vi "Camera.v10.vi"() -> ()   [LabVIEW 2015]
uses:
  Camera Properties.ctl
  Microscope Settings.ctl
  CameraState.ctl
  ModeEnum.ctl
  Stack_State.ctl
  Stack Track.ctl
  CameraControlTypeDef.ctl
  <vilib>/DAQmx/write.llb/DAQmx Write (Digital 1D Wfm NChan NSamp).vi
  <vilib>/DAQmx/write.llb/DAQmx Write (Analog 1D Wfm NChan NSamp).vi
  <vilib>/DAQmx/create/channels.llb/DAQmx Create Channel (DO-Digital Output).vi
  <vilib>/DAQmx/create/channels.llb/DAQmx Create Channel (AO-Voltage-Basic).vi
  <vilib>/Waveform/DWDTOps.llb/DWDT Append Digital Samples.vi
  <vilib>/Waveform/WDTOps.llb/WDT Append Waveforms DBL.vi
  <vilib>/Waveform/WDTOps.llb/WDT Number of Waveform Samples DBL.vi
  <vilib>/DAQmx/configure/timing.llb/DAQmx Timing (Sample Clock).vi
  <vilib>/Waveform/DWDTOps.llb/DWDT Uncompress Digital.vi
  <vilib>/DAQmx/miscellaneous.llb/DAQmx Fill In Error Info.vi
  <vilib>/vision/NI_Vision_Development_Module.lvlib
panel:
  in  "Tab Control":enum32{"Camera Settings", "Recording"}(tab)
  in  "Scans":dbl=1.0 min=0.0 max=10.0 step=0.05
  in  "?":bool
  in  "Microscope Settings":T1={"Mode"=enum."XY", "Slit"={"Scanning Mode"=12.0, "Slit Width /%"=5.0}, "Colour"=[{"Laser"=enum."561", "Filter"=4}], "Exposure/ms"=40.0, "Piezo Position /um"=0.0, "ROI"={"X"={"Start"=0.0, "Step"=1.0, "Range"=2048.0}, "Y"={"Start"=0.0, "Step"=1.0, "Range"=2048.0}, "Z "={"Start"=0.0, "Step"=1.0, "Range"=100.0}}, "Samples per millisecond"=100.0, "Relax/ms"=10.0, "Readout Direction"=2.0, "Trigger Source"=2.0, "Camera Delay /ms"=11.0, "Under Scan"=5.0} {"Under Scan" min=0.0 max=10.0 step=0.05; "ROI"."X"."Range" min=0.0 max=10.0 step=0.05; "ROI"."X"."Step" min=0.0 max=10.0 step=0.05; "ROI"."X"."Start" min=0.0 max=10.0 step=0.05; "ROI"."Y"."Range" min=0.0 max=10.0 step=0.05; "ROI"."Y"."Step" min=0.0 max=10.0 step=0.05; "ROI"."Y"."Start" min=0.0 max=10.0 step=0.05; "ROI"."Z"."Range" min=0.0 max=10.0 step=0.05; "ROI"."Z"."Step" min=0.0 max=10.0 step=0.05; "ROI"."Z"."Start" min=0.0 max=10.0 step=0.05; "Colour"."Filter" items=["Empty"=1, ""=2, ""=3, "561"=4, ""=5, "488"=6]; "Camera Delay /ms" min=0.0 max=10.0 step=0.05; "Trigger Source" items=["Internal"=1.0, "External"=2.0]; "Readout Direction" items=["Forward"=1.0, "Backward"=2.0]; "Slit"."Scanning Mode" items=["Full Frame"=1.0, "Slit Scanning"=12.0]; "Piezo Position /um" min=0.0 max=10.0 step=0.05}
  in  "Scan":bool
  in  "Scan Continuously":bool
  out "error IO":errorcluster
  in  "Advanced DCAM Controls":i32(listbox) caption="Multicolumn Listbox"
  in  "Properties":T2=4211904 items=["SENSOR MODE"=4212128, "CCD MODE"=4212384, "READOUT MODE"=4211872, "ACTIVE VIEW INDEX"=4343136, "BITS PER CHANNEL"=4342976, "IMAGE PIXEL TYPE"=4343296, "BINNING"=4215968, "EXPOSURE TIME"=2049184, "CONTRAST GAIN"=3163312, "CONTRAST OFFSET"=3163328, "LIGHT MODE"=2114720, "SENSITIVITY"=2114992, "PHOTON IMAGING MODE"=2115200, "HIGH DYNAMIC RANGE MODE"=3163360, "WHITE BALANCE"=3163568, "TEMPERATURE"=2115232, "TEMPERATURE TARGET"=2115264, "SENSOR COOLER FAN"=2115296, "LINEBUNDLE HEIGHT"=4212192, "MECHANICAL SHUTTER"=2115488, "BACK FOCUS POSITION"=8422304, "TRIGGER CONNECTOR"=1066432, "TRIGGER SOURCE"=1066144, "OUTPUT TRIGGER SOURCE"=1852576, "TRIGGER GLOBAL EXPOSURE"=2049680, "FIRST TRIGGER BEHAVIOR"=2049696, "CHANNEL SYNC"=1852352, "READOUT DIRECTION"=4211904, "PRE HSYNC COUNT"=1852704, "INTERNAL LINE SPEED"=4191408, "INTERNAL LINE INVERVAL"=4191424]
  in  "Multicolumn Listbox":i32(listbox)
  out "Image":T3(plugin-control)
  out "Histogram":T4(graph)
  in  "stop":bool
  in  "Signals Debugger":bool
  in  "Calibration":bool
  in  "MultiD Scan":bool
  in  "Stage Controller":bool
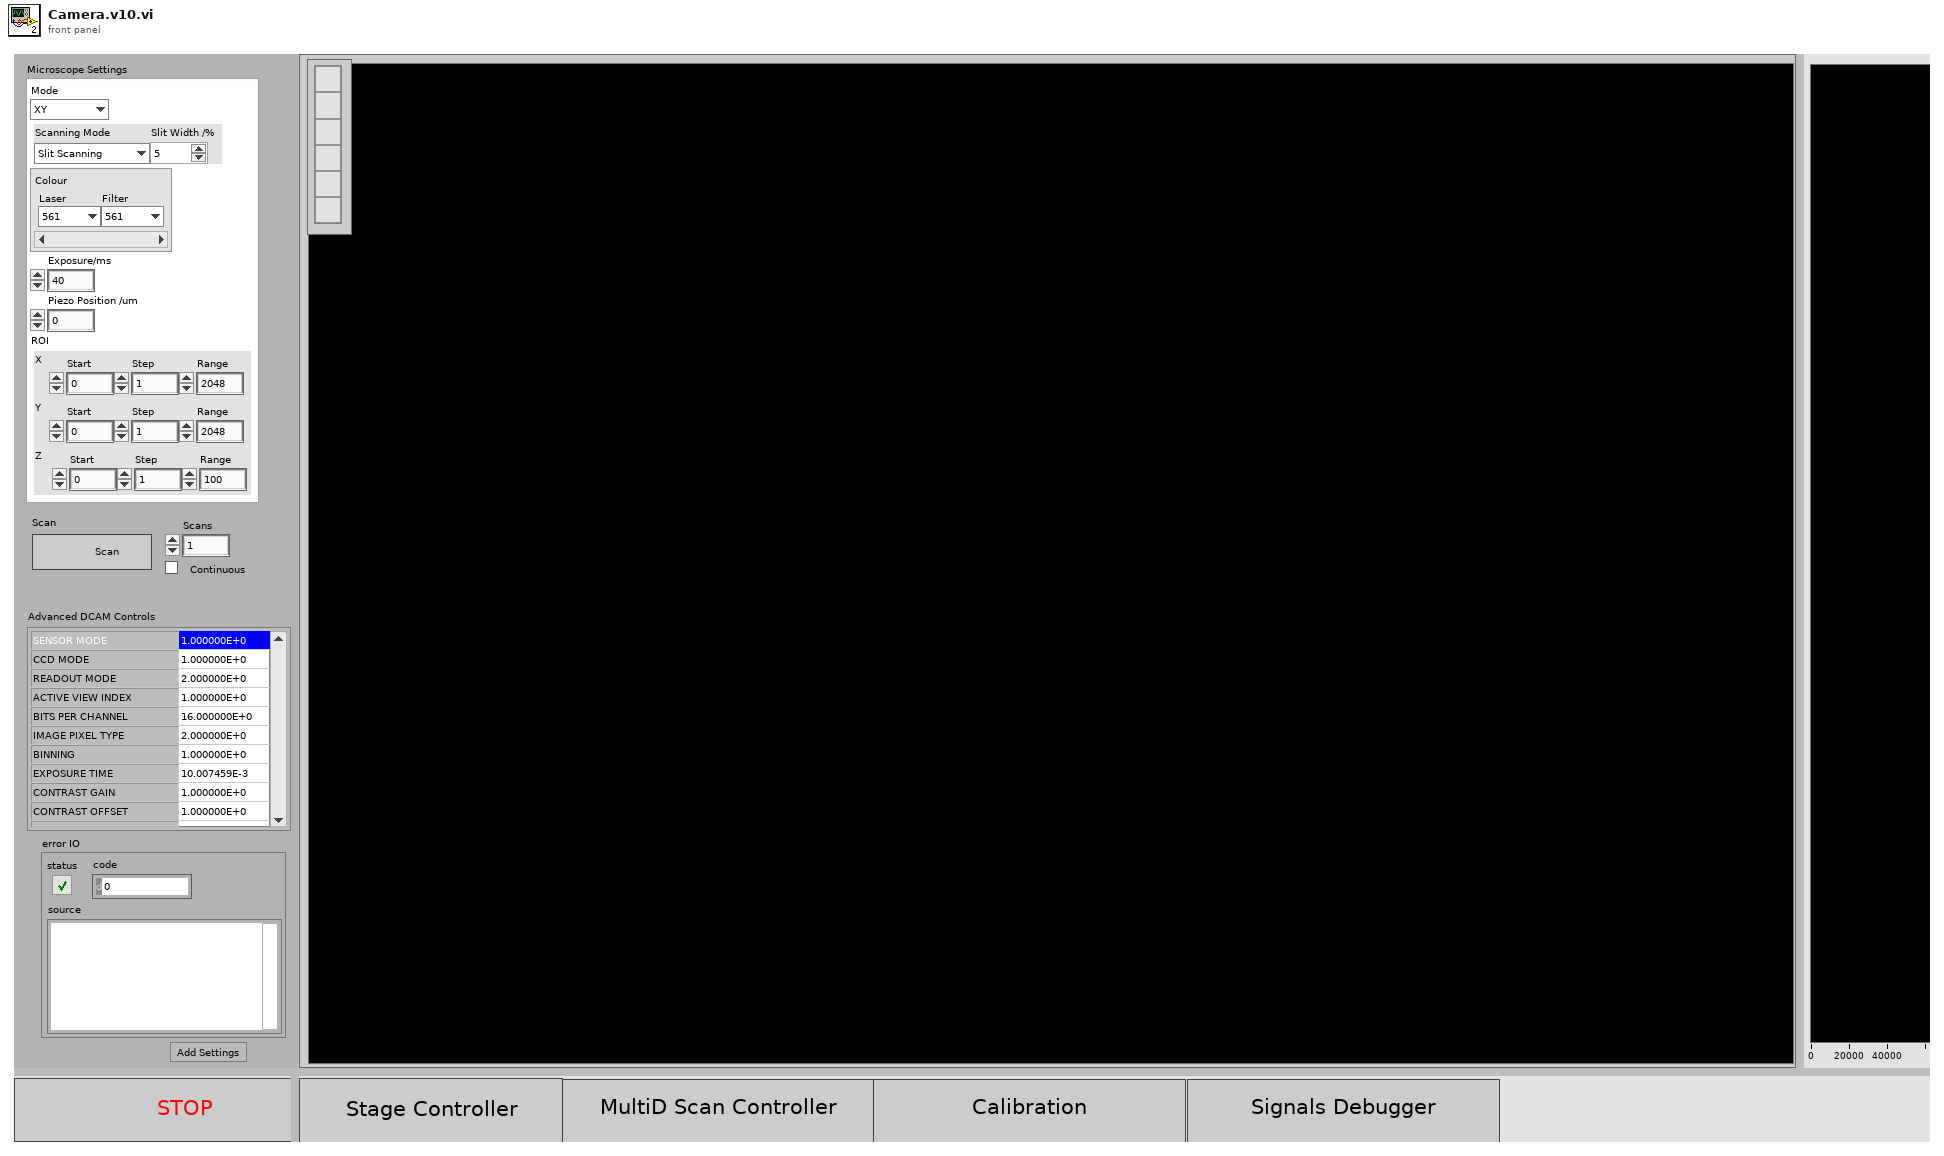
[diagram p1: front panel]
types:
  T1 = typedef "Microscope Settings.ctl" = cluster{"Mode":enum16{"X", "XY", "XYZ", "XYZT", "XYZC"}, "Slit":cluster{"Scanning Mode":dbl, "Slit Width /%":dbl}, "Colour":cluster{"Laser":enum16{"Brightfield", "445", "488", "561", "647"}, "Filter":u16}[], "Exposure/ms":dbl, "Piezo Position /um":dbl, "ROI":cluster{"X":cluster{"Start":dbl, "Step":dbl, "Range":dbl}, "Y":cluster{"Start":dbl, "Step":dbl, "Range":dbl}, "Z ":cluster{"Start":dbl, "Step":dbl, "Range":dbl}}, "Samples per millisecond":dbl, "Relax/ms":dbl, "Readout Direction":dbl, "Trigger Source":dbl, "Camera Delay /ms":dbl, "Under Scan":dbl}
  T2 = typedef "Camera Properties.ctl" = u32
  T3 = typedef "IMAQ Image.ctl" = refnum<image>
  T4 = cluster{"Starting Value":sgl, "Incremental Value":sgl, "Histogram":u32[]}
  T5 = cluster{"height":u32, "width":u32, "datatype":u32}
  T6 = typedef "CameraState.ctl" = enum16{"init", "active", "deinit"}
  T7 = typedef "ModeEnum.ctl" = enum16{"Idle", "generateWaves", "runWaves", "stop"}
  T8 = typedef "CameraControlTypeDef.ctl" = enum16{"Idle", "IntervalLineInt", "Ram Record", "HardDisk Record", "Disengage Update", "Update", "ROI", "Binning", "Scan Mode", "Trigger Mode", "Readout Mode", "Readout Direction", "Preview", "ROIWindow", "Trigger Source"}
  T9 = cluster{"Mode":u32, "Polarity":u32, "Times":u32, "Delay":dbl}
  T10 = typedef "Stack_State.ctl" = cluster{"State":T11, "Stack Number":i32, "Image":u16[][], "Stacks":i32}
  T11 = typedef "Stack Track.ctl" = enum16{"Idle", "Display", "Start Sequence", "Read Disk", "STOP", "Collecting", "End"}
  T12 = enum32{"Invalid", "Standard", "Closed", "Hidden", "Minimized", "Maximized"}
  T13 = typedef "Image Type" = u32
  T14 = cluster{"Analogue Out":waveform(dbl)[], "Digital Out":digitalwaveform[]}
  T15 = cluster{"State":T11, "Timeout":i32, "Data 16":u16[][], "Timeout":i32}
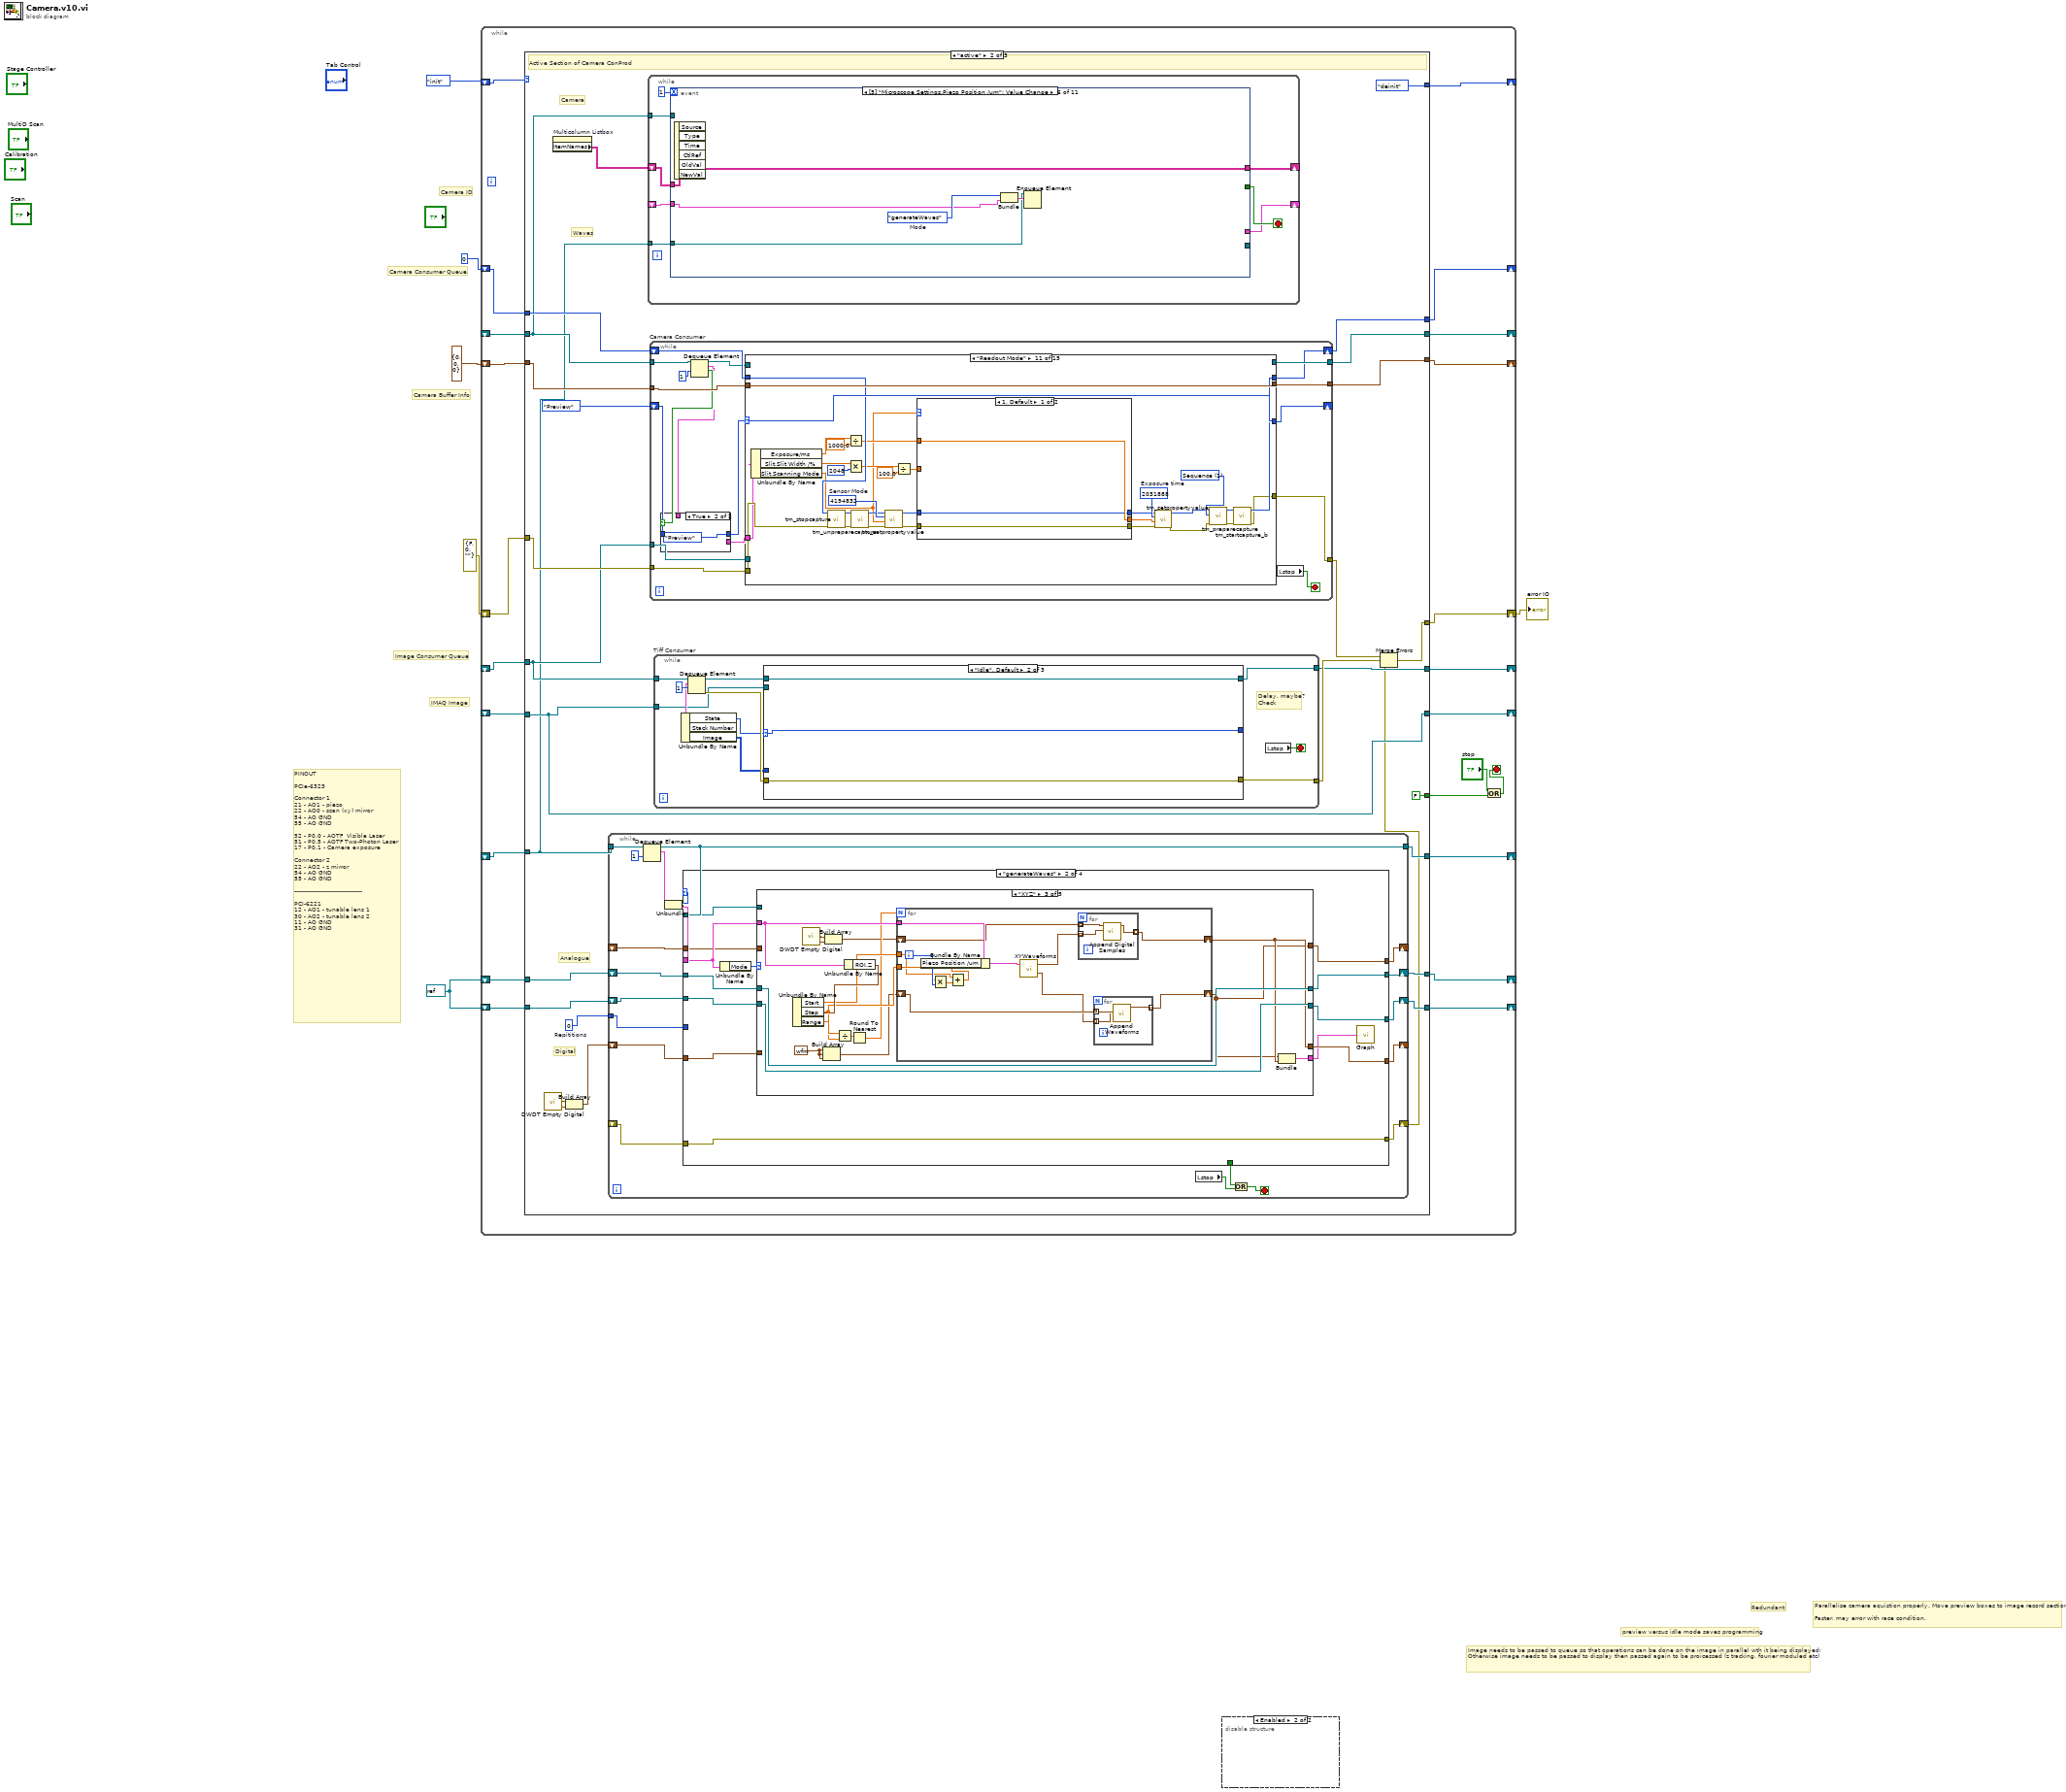
[diagram p0: block diagram]
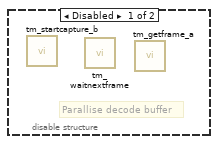
[diagram p2: hidden frame]
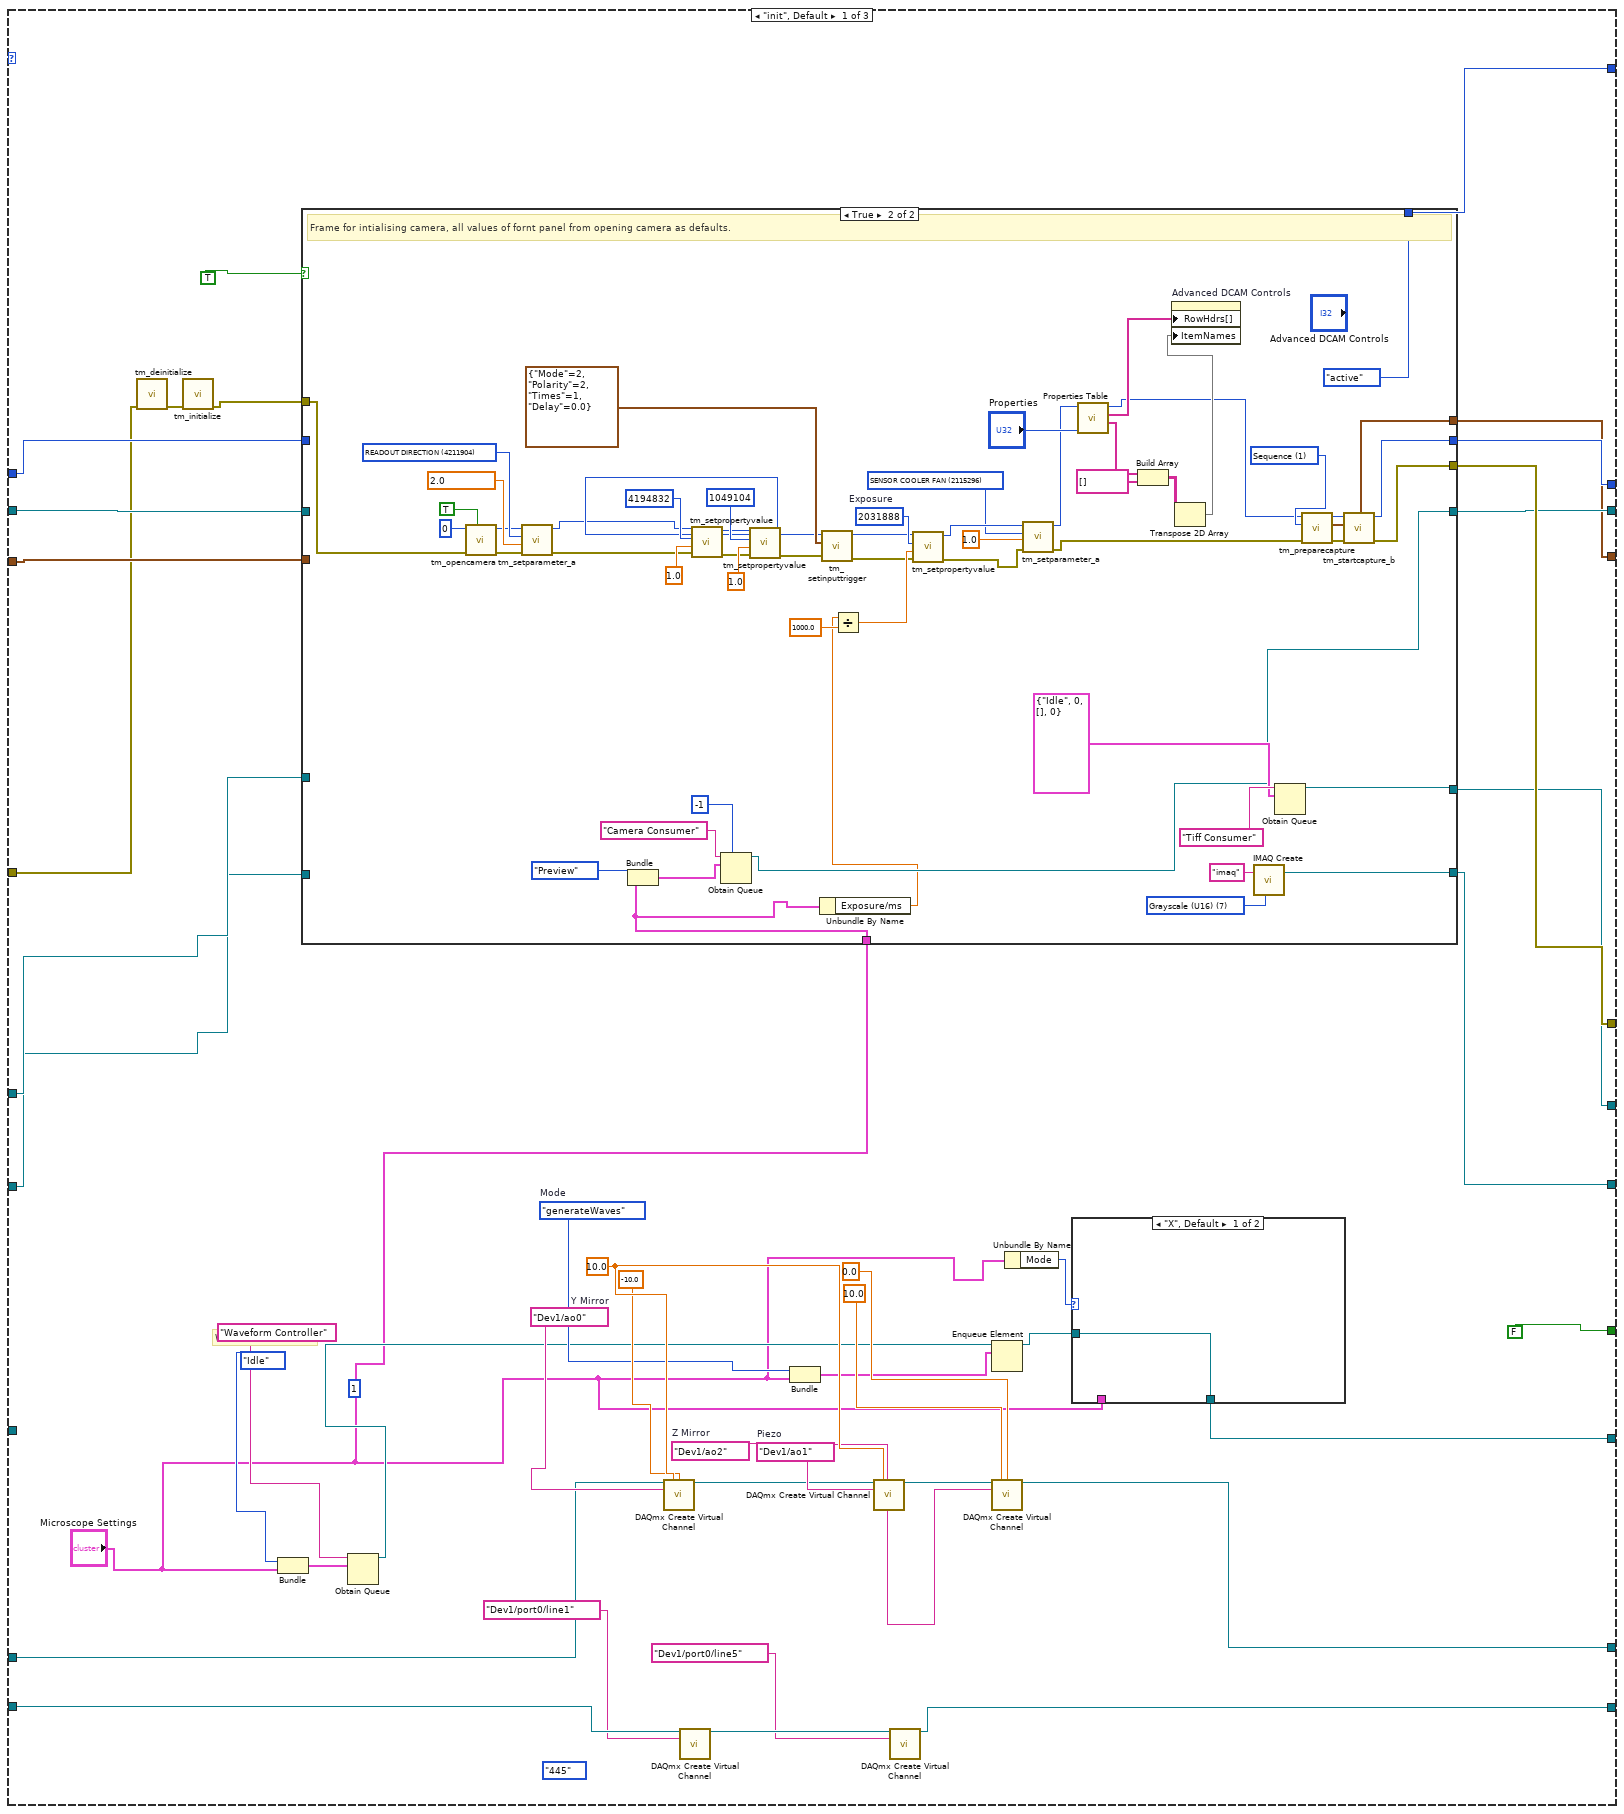
[diagram p3: hidden frame]
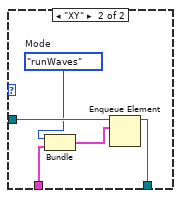
[diagram p4: hidden frame]
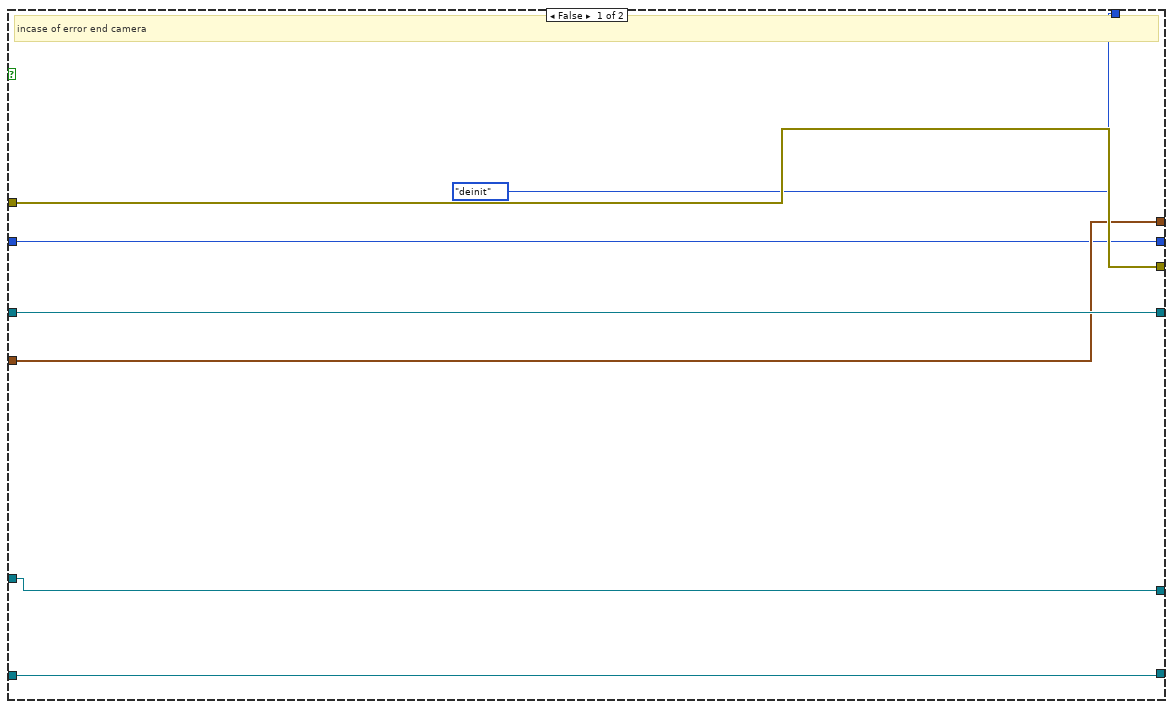
[diagram p5: hidden frame]
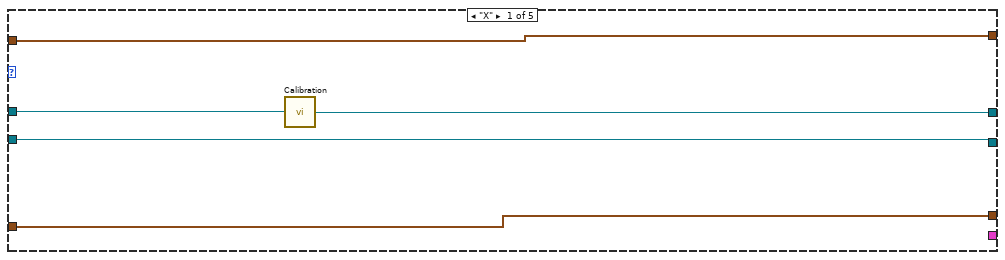
[diagram p7: hidden frame]
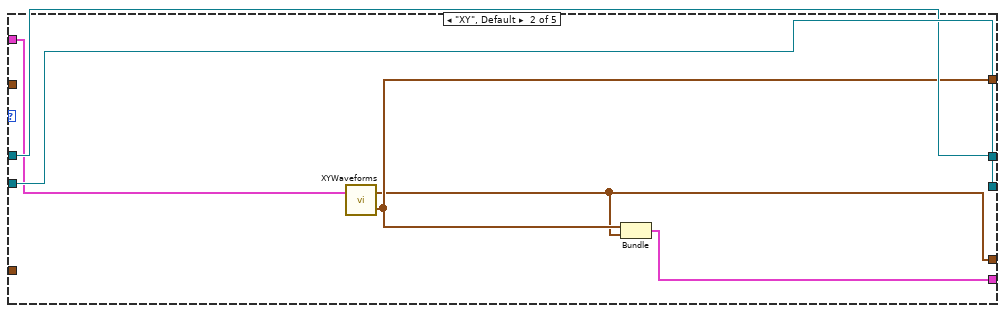
[diagram p8: hidden frame]
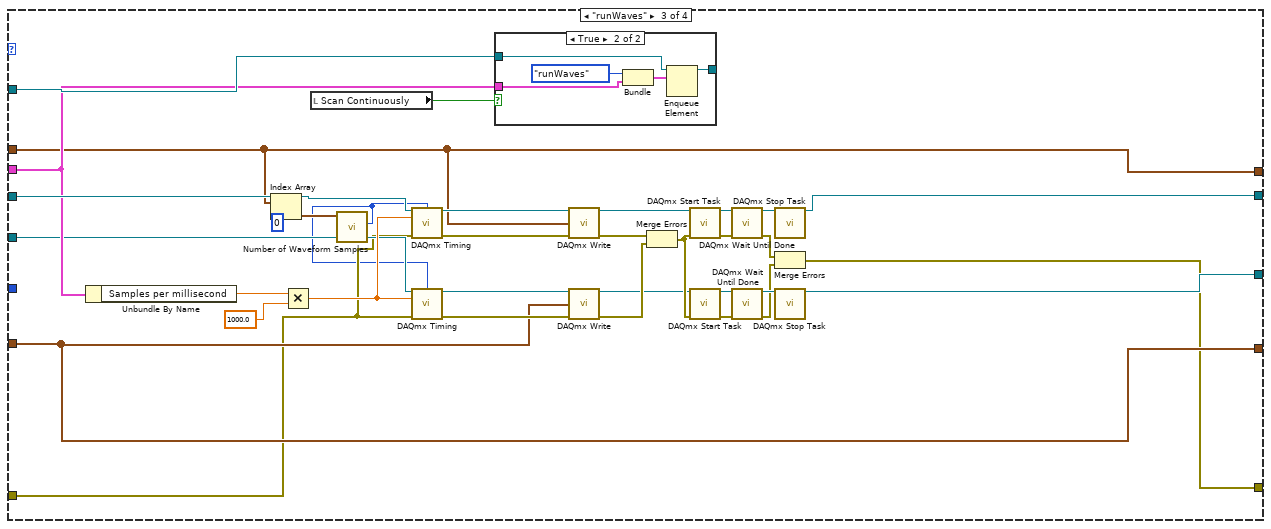
[diagram p11: hidden frame]
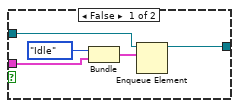
[diagram p12: hidden frame]
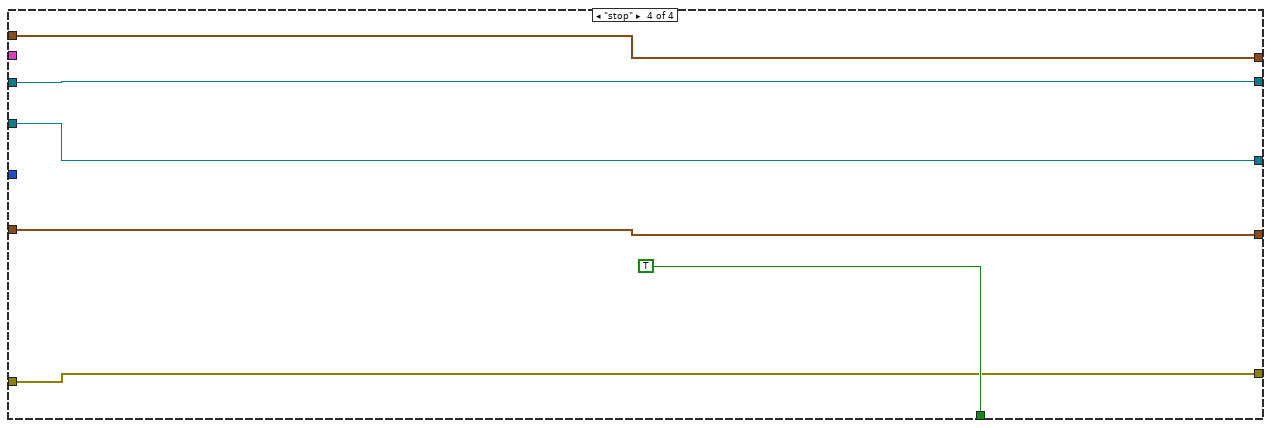
[diagram p13: hidden frame]
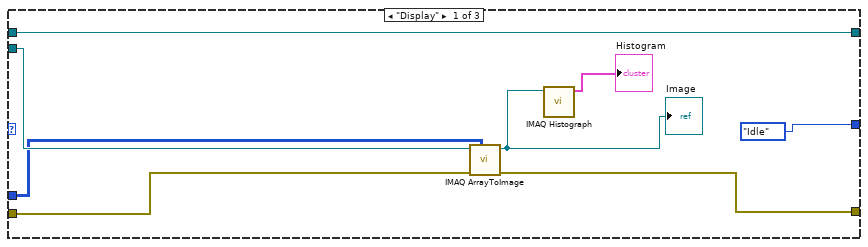
[diagram p14: hidden frame]
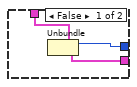
[diagram p16: hidden frame]
diagram:
  w3 = refnum<k21> refnum ("Mirror Z 2")
  # "PINOUT\n\nPCIe-6323\n\nConnector 1\n21 - AO1 - piezo\n22 - AO0 - scan (xy) mirror\n54 - AO GND\n55 - AO GND\n\n52 - P0.0 - AOTF  Visible Laser\n51 - P0.5 - AOTF Two-Photon Laser\n17 - P0.1 - Camera exposure\n\nConnector 2\n22 - AO2 - z mirror\n54 - AO GND\n55 - AO GND\n\n-----------------------------------\n\nPCI-6221\n12 - AO1 - tunable lens 1\n30 - AO2 - tunable lens 2\n11 - AO GND\n31 - AO GND"
  # "IMAQ Image"
  # "Camera Buffer Info"
  # "Image needs to be passed to queue so that operations can be done on the image in parallel wth it being displayed;\nOtherwise image needs to be passed to display then passed again to be proicessed (z tracking, fourier moduled etc)"
  # "preview versus idle mode saves programming"
  # "Parallelise camera aquistion properly. Move preview boxes to image record section.\n\nFaster. may error with race condition."
  # "Redundant"
  # "Image Consumer Queue"
  # "Camera Consumer Queue"
  # "Camera ID"
  n1 = while {
    shift-right: [w29] -> _
    shift-left: CameraState."init" -> [w28]
    shift-right: [w27] -> _
    shift-left: u32 0 ("Handle out") -> [w26]
    shift-right: [w25] -> w5
    shift-left: errorcluster {"status"=FALSE, "code"=0, "source"=""} ("error IO") -> [w24]
    shift-right: [w22] -> _
    shift-left: _ -> [w21]
    shift-right: [w23] -> _
    shift-left: _ -> [w20]
    shift-right: [w16] -> _
    shift-left: T5 {"height"=0, "width"=0, "datatype"=0} ("Buffer Info") -> [w15]
    shift-right: [w14] -> _
    shift-left: _ -> [w13]
    shift-right: [w12] -> _
    shift-left: w3 -> [w11]
    shift-right: [w9] -> _
    shift-left: w3 -> [w10]
    shift-right: [w8] -> _
    shift-left: _ -> [w7]
    stop <- w18 stop-if-true
    n2 = case shown="\"active\"" w28 {
      tunnel: [w70 CameraState."deinit" CameraState."init"] -> w29
      tunnel: [w69 w167 w627] -> w27
      tunnel: w26 -> [w47 w168 w627]
      tunnel: [w68 w166 w630] -> w25
      tunnel: w24 -> [w46 w160 w631]
      tunnel: [w67 w163 w614] -> w23
      tunnel: [w66 w162 w610] -> w22
      tunnel: w21 -> [w64 w155 w610]
      tunnel: w20 -> [w65 w153 w614]
      tunnel: [FALSE ("stop") FALSE ("stop") TRUE ("stop")] -> w17
      tunnel: [w62 w158 w624] -> w16
      tunnel: w15 -> [w61 w157 w624]
      tunnel: w13 -> [w59 w154 w623]
      tunnel: [w60 w154 w623] -> w14
      tunnel: w7 -> [_ w145 w609]
      tunnel: [w51 w146 w621] -> w12
      tunnel: w11 -> [w48 w149 w621]
      tunnel: w10 -> [w44 w148 w619]
      tunnel: [w39 w147 w619] -> w9
      tunnel: [w35 w144 w609] -> w8
      frame "init", Default {
        (unwired) enum16{"445", "488", "561", "647"}."445" ("Laser")
        (unwired) 1 ("max queue size (-1, unlimited)")
        w43 = ModeEnum."generateWaves"  # Mode
        w54 = tag "Dev1/ao1"  # Piezo
        w55 = tag "Dev1/ao2"  # Z Mirror
        w56 = tag "Dev1/ao0"  # Y Mirror
        w58 = 10.0 ("maximum value")
        # "Waveform controls"
        n3 = call "tm_deinitialize.vi"("error in (no error)"=w46) -> ("error out"=w72:errorcluster)  [unwired: 10 in]
        n4 = call "tm_initialize.vi"("error in (no error)"=w72) -> ("error out"=w71:errorcluster)  [unwired: 7 in, 3 out]
        n5 = Bundle("Mode"=ModeEnum."Idle", "Microscope Settings"="Microscope Settings") -> (w41:cluster{"Mode":T7, "Microscope Settings":T1})  [unwired: 1 in]
        n6 = case shown="True" TRUE {
          tunnel: w71 -> [w85 w106]
          tunnel: [CameraState."deinit" CameraState."active"] -> w70
          tunnel: [w85 w137] -> w68
          tunnel: [w80 w135] -> w69
          tunnel: [w83 w125] -> w67
          tunnel: [w82 w132] -> w66
          tunnel: w65 -> [w83 _]
          tunnel: w64 -> [w82 _]
          tunnel: [w81 w130] -> w62
          tunnel: w61 -> [w81 _]
          tunnel: w47 -> [w80 _]
          tunnel: [w79 w127] -> w60
          tunnel: w59 -> [w79 _]
          tunnel: "Microscope Settings" -> [_ w93]
          frame False {
            # "incase of error end camera"
          }
          frame True {
            w103 = u32 2115296 items=["SENSOR MODE"=4212128, "CCD MODE"=4212384, "READOUT MODE"=4211872, "ACTIVE VIEW INDEX"=4343136, "BITS PER CHANNEL"=4342976, "IMAGE PIXEL TYPE"=4343296, "BINNING"=4215968, "EXPOSURE TIME"=2049184, "CONTRAST GAIN"=3163312, "CONTRAST OFFSET"=3163328, "LIGHT MODE"=2114720, "SENSITIVITY"=2114992, "PHOTON IMAGING MODE"=2115200, "HIGH DYNAMIC RANGE MODE"=3163360, "WHITE BALANCE"=3163568, "TEMPERATURE"=2115232, "TEMPERATURE TARGET"=2115264, "SENSOR COOLER FAN"=2115296, "LINEBUNDLE HEIGHT"=4212192, "MECHANICAL SHUTTER"=2115488, "BACK FOCUS POSITION"=8422304, "TRIGGER CONNECTOR"=1066432, "TRIGGER SOURCE"=1066144, "OUTPUT TRIGGER SOURCE"=1852576, "TRIGGER GLOBAL EXPOSURE"=2049680, "FIRST TRIGGER BEHAVIOR"=2049696, "CHANNEL SYNC"=1852352, "READOUT DIRECTION"=4211904, "PRE HSYNC COUNT"=1852704, "INTERNAL LINE SPEED"=4226000, "INTERNAL LINE INTERVAL"=4226016] ("Parameter")
            w112 = u32 2031888  # Exposure
            w123 = sgl 2.0 items=["Forward"=1.0, "Backward"=2.0] ("Readout Direction")
            w124 = u32 4211904 items=["SENSOR MODE"=4212128, "CCD MODE"=4212384, "READOUT MODE"=4211872, "ACTIVE VIEW INDEX"=4343136, "BITS PER CHANNEL"=4342976, "IMAGE PIXEL TYPE"=4343296, "BINNING"=4215968, "EXPOSURE TIME"=2049184, "CONTRAST GAIN"=3163312, "CONTRAST OFFSET"=3163328, "LIGHT MODE"=2114720, "SENSITIVITY"=2114992, "PHOTON IMAGING MODE"=2115200, "HIGH DYNAMIC RANGE MODE"=3163360, "WHITE BALANCE"=3163568, "TEMPERATURE"=2115232, "TEMPERATURE TARGET"=2115264, "SENSOR COOLER FAN"=2115296, "LINEBUNDLE HEIGHT"=4212192, "MECHANICAL SHUTTER"=2115488, "BACK FOCUS POSITION"=8422304, "TRIGGER CONNECTOR"=1066432, "TRIGGER SOURCE"=1066144, "OUTPUT TRIGGER SOURCE"=1852576, "TRIGGER GLOBAL EXPOSURE"=2049680, "FIRST TRIGGER BEHAVIOR"=2049696, "CHANNEL SYNC"=1852352, "READOUT DIRECTION"=4211904, "PRE HSYNC COUNT"=1852704, "INTERNAL LINE SPEED"=4226000, "INTERNAL LINE INTERVAL"=4226016] ("Parameter")
            w129 = T13 7 items=["Grayscale (U8)", "Grayscale (I16)", "Grayscale (SGL)", "Complex (CSG)", "RGB (U32)", "HSL (U32)", "RGB (U64)", "Grayscale (U16)"] ("Image Type")
            w139 = 1 items=["Snap", "Sequence"] ("Capture mode")
            # "Frame for intialising camera, all values of fornt panel from opening camera as defaults."
            n7 = call "tm_opencamera.vi"("Force Open"=TRUE, "error in (no error)"=w106, "Camera Index"=u32 0) -> ("error out"=w121:errorcluster, "Handle out"=w122:u32)  [unwired: 6 in, 1 out]
            n8 = call "tm_setparameter_a.vi"("error in (no error)"=w121, "Value in"=w123, "Parameter"=w124, "Handle in"=w122) -> ("error out"=w91:errorcluster, "Handle out"=w113:u32)  [unwired: 6 in]
            n9 = Bundle("Enum"=CameraControlTypeDef."Preview", "Microscope Settings"=w93) -> (w107:cluster{"Enum":T8, "Microscope Settings":T1})  [unwired: 1 in]
            n10 = call "tm_setpropertyvalue.vi"("error in (no error)"=w91, "Value in"=sgl 1.0, "Property ID"=u32 4194832, "Handle in"=w113) -> ("error out"=w90:errorcluster, "Handle out"=w116:u32)  [unwired: 6 in]
            n11 = Obtain Queue(max queue size (-1, unlimited)=-1, name (unnamed)="Camera Consumer", element data type=w107) -> (queue out=w125:refnum<queue>)  [unwired: 2 in, 2 out]
            n12 = call "tm_setpropertyvalue.vi"("error in (no error)"=w90, "Value in"=sgl 1.0, "Property ID"=u32 1049104, "Handle in"=w116) -> ("error out"=w89:errorcluster, "Handle out"=w114:u32)  [unwired: 6 in]
            n13 = Unbundle By Name(w93) -> ("Exposure/ms"=w92:dbl)
            n14 = call <userlib>:"tm_setinputtrigger.vi"("error in (no error)"=w89, "Parameters"=T9 {"Mode"=2, "Polarity"=2, "Times"=1, "Delay"=0.0}, "Handle in"=w114) -> ("error out"=w88:errorcluster, "Handle out"=w111:u32)  [unwired: 7 in]
            n15 = Divide(x=w92, y=sgl 1000.0) -> (x/y=w109:dbl)
            n16 = call "tm_setpropertyvalue.vi"("error in (no error)"=w88, "Value in"=w109, "Property ID"=w112, "Handle in"=w111) -> ("error out"=w87:errorcluster, "Handle out"=w104:u32)  [unwired: 6 in]
            n17 = call "tm_setparameter_a.vi"("error in (no error)"=w87, "Value in"=1.0, "Parameter"=w103, "Handle in"=w104) -> ("error out"=w86:errorcluster, "Handle out"=w95:u32)  [unwired: 6 in]
            n18 = call "Properties Table.vi"("Properties"="Properties", "Handle In"=w95) -> ("Value Stirngs Out"=w99:string[], "Row Headers"=w100:string[], "Handle Out"=w94:u32)  [unwired: 3 in, 1 out]
            n19 = Build Array(w99, string[] [] ("element")) -> (w97:string[][])
            n20 = Transpose 2D Array(2D array=w97) -> (transposed array=w96:string[][])
            n21 = property on="Advanced DCAM Controls" class="MCListbox (strict)"("RowHdrs[]"=w100, "ItemNames"=w96) -> ()  [unwired: 2 in, 2 out]
            n22 = call "IMAQ Create"("Image Name"="imaq", "Image Type"=w129) -> ("New Image"=w127:T3)  [unwired: 3 in, 1 out]
            n23 = Obtain Queue(name (unnamed)="Tiff Consumer", element data type=T10 {"State"=enum."Idle", "Stack Number"=0, "Image"=[], "Stacks"=0} ("input cluster")) -> (queue out=w132:refnum<queue>)  [unwired: 3 in, 2 out]
            n24 = call "tm_preparecapture.vi"("error in (no error)"=w86, "Capture mode"=w139, "Handle in"=w94) -> ("error out"=w138:errorcluster, "Buffer Info"=w130:T5, "Handle out"=w136:u32)  [unwired: 5 in, 1 out]
            n25 = call "tm_startcapture_b.vi"("error in (no error)"=w138, "Handle in"=w136) -> ("error out"=w137:errorcluster, "Handle out"=w135:u32)  [unwired: 8 in]
          }
        }
        n26 = Obtain Queue(name (unnamed)="Waveform Controller", element data type=w41) -> (queue out=w40:refnum<queue>)  [unwired: 3 in, 2 out]
        n27 = call-poly <vilib>:"DAQmx Create Virtual Channel.vi"("task in"=w48, "maximum value"=w58, "minimum value"=-10.0, "physical channels"=w56) -> ("task out"=w50:refnum<k21>)  [unwired: 10 in, 1 out]
        n28 = call-poly <vilib>:"DAQmx Create Virtual Channel.vi"("task in"=w44, "lines"=tag "Dev1/port0/line1") -> ("task out"=w45:refnum<k21>)  [unwired: 12 in, 1 out]
        n29 = Bundle("Mode"=w43, "Microscope Settings"="Microscope Settings") -> (w32:cluster{"Mode":T7, "Microscope Settings":T1})  [unwired: 1 in]
        n30 = call-poly <vilib>:"DAQmx Create Virtual Channel.vi"("task in"=w50, "maximum value"=w58, "physical channels"=w55) -> ("task out"=w49:refnum<k21>)  [unwired: 11 in, 1 out]
        n31 = call-poly <vilib>:"DAQmx Create Virtual Channel.vi"("task in"=w45, "lines"=tag "Dev1/port0/line5") -> ("task out"=w39:refnum<k21>)  [unwired: 12 in, 1 out]
        n32 = Enqueue Element(queue=w40, element=w32) -> (queue out=w36:refnum<queue>)  [unwired: 2 in, 2 out]
        n33 = call-poly <vilib>:"DAQmx Create Virtual Channel.vi"("task in"=w49, "maximum value"=10.0 ("minimum value"), "minimum value"=0.0 ("maximum value"), "physical channels"=w54) -> ("task out"=w51:refnum<k21>)  [unwired: 10 in, 1 out]
        n34 = Unbundle By Name("Microscope Settings") -> ("Mode"=w31:enum16{"X", "XY", "XYZ", "XYZT", "XYZC"})
        n35 = case shown="\"X\", Default" w31 {
          tunnel: w36 -> [w73 w78]
          tunnel: [w73 w76] -> w35
          tunnel: "Microscope Settings" -> [_ w75]
          frame "X", Default {
          }
          frame "XY" {
            w74 = ModeEnum."runWaves"  # Mode
            n36 = Bundle("Mode"=w74, "Microscope Settings"=w75) -> (w77:cluster{"Mode":T7, "Microscope Settings":T1})  [unwired: 1 in]
            n37 = Enqueue Element(queue=w78, element=w77) -> (queue out=w76:refnum<queue>)  [unwired: 2 in, 2 out]
          }
        }
      }
      frame "active" {
        w152 = 0  # Repititions
        # "Waves"
        # "Camera"
        # "Digital"
        # "Analogue"
        # "Active Section of Camera ConProd"
        n38 = call <vilib>:"DWDT Empty Digital.vi"() -> ("digital waveform out"=w150:digitalwaveform)  [unwired: 5 in]
        n39 = property on="Multicolumn Listbox" class="MCListbox (strict)"() -> ("ItemNames"=w142:string[][])  [unwired: 2 in, 2 out]
        n40 = Build Array(w150, w150) -> (w151:digitalwaveform[])
        n41 = while {
          tunnel: w145 -> [w188]
          shift-right: [w184] -> _
          shift-left: _ -> [w183]
          tunnel: w152 -> [w182]
          shift-right: [w178] -> w146
          shift-left: w149 -> [w177]
          shift-right: [w181] -> _
          shift-left: w151 -> [w180]
          shift-right: [w176] -> w147
          shift-left: w148 -> [w175]
          tunnel: [w174] -> w144
          shift-right: [w173] -> w143
          shift-left: _ -> [w172]
          stop <- w169 stop-if-true
          n42 = Dequeue Element(queue=w188, timeout in ms (-1)=1) -> (queue out=w174:refnum<queue>, element=w187:cluster{"Mode":T7, "Microscope Settings":T1})  [unwired: 1 in, 2 out]
          n43 = Unbundle(w187) -> ("Mode"=w186:T7, "Microscope Settings"=w185:T1)
          n44 = case shown="\"generateWaves\"" w186 {
            tunnel: [_ _ _ TRUE] -> w171
            tunnel: w185 -> [_ w205 w289 _]
            tunnel: [w193 w206 w288 w310] -> w184
            tunnel: w183 -> [w193 w197 w288 w310]
            tunnel: w182 -> [_ _ _ _]
            tunnel: w174 -> [_ w196 w290 _]
            tunnel: [w190 w201 w268 w309] -> w176
            tunnel: [w191 w199 w283 w308] -> w178
            tunnel: w177 -> [w191 w198 w291 w308]
            tunnel: [w192 w204 w270 w307] -> w181
            tunnel: w180 -> [w192 w203 w270 w307]
            tunnel: w175 -> [w190 w202 w279 w309]
            tunnel: [w189 w195 w265 w305] -> w173
            tunnel: w172 -> [w189 w195 w264 w305]
            frame "Idle", Default {
            }
            frame "generateWaves" {
              n45 = Unbundle By Name(w205) -> ("Mode"=w200:enum16{"X", "XY", "XYZ", "XYZT", "XYZC"})
              n46 = case shown="\"XYZ\"" w200 {
                tunnel: [w211 w214 w222 w256 w260] -> w206
                tunnel: w205 -> [_ w215 w233 _ _]
                tunnel: [w209 w213 w226 w253 w257] -> w204
                tunnel: w203 -> [w209 _ _ w253 w257]
                tunnel: w202 -> [w210 w217 w227 w254 w258]
                tunnel: [w210 w217 w227 w254 w258] -> w201
                tunnel: [w207 w216 w228 w255 w259] -> w199
                tunnel: w198 -> [w208 w216 w228 w255 w259]
                tunnel: w197 -> [w211 _ _ w256 w260]
                tunnel: w196 -> [_ _ _ _ _]
                tunnel: [_ w212 w223 _ _] -> w194
                frame "X" {
                  n47 = call "Calibration.vi"("Analogue In"=w208) -> ("Analogue In Out"=w207:refnum<k21>)
                }
                frame "XY", Default {
                  n48 = call "XYWaveforms.vi"("Microscope Settings"=w215) -> ("Analogue Out"=w214:waveform(dbl)[], "Digital Out"=w213:digitalwaveform[])  [unwired: 1 in]
                  n49 = Bundle("Analogue Out"=w214, "Digital Out"=w213) -> (w212:T14)  [unwired: 1 in]
                }
                frame "XYZ" {
                  w218 = waveform(dbl) {"t0"=timestamp(0 s since 1904-01-01), "dt"=1.0, "Y"=[]} ("Waveform")
                  n50 = call <vilib>:"DWDT Empty Digital.vi"() -> ("digital waveform out"=w221:digitalwaveform)  [unwired: 5 in]
                  n51 = Build Array(w218, w218, w218) -> (w219:waveform(dbl)[])
                  n52 = Build Array(w221, w221) -> (w220:digitalwaveform[])
                  n53 = Unbundle By Name(w233) -> ("ROI.Z"=w232:cluster{"Start":dbl, "Step":dbl, "Range":dbl})
                  n54 = Unbundle By Name(w232) -> ("Start"=w231:dbl, "Step"=w229:dbl, "Range"=w230:dbl)
                  n55 = Divide(x=w230, y=w229) -> (x/y=w225:dbl)
                  n56 = Round To Nearest(number=w225) -> (nearest integer value=w224:dbl)
                  n57 = for {
                    N: w224 -> [_]
                    tunnel: w233 -> [w246]
                    tunnel: w229 -> [w242]
                    tunnel: w231 -> [w241]
                    shift-right: [w237] -> w222
                    shift-left: w219 -> [w239]
                    shift-right: [w235] -> w226
                    shift-left: w220 -> [w234]
                    i -> [w243]
                    n58 = Multiply(x=w242, y=w243) -> (x*y=w244:dbl)
                    n59 = Add(x=w241, y=w244) -> (x+y=w240:dbl)
                    n60 = Bundle By Name(cluster=w246, "Piezo Position /um"=w240) -> (w245:T1)
                    n61 = call "XYWaveforms.vi"("Microscope Settings"=w245) -> ("Analogue Out"=w238:waveform(dbl)[], "Digital Out"=w236:digitalwaveform[])  [unwired: 1 in]
                    n62 = for {
                      tunnel: w236 -> [w248] mode=indexing
                      tunnel: w234 -> [w249] mode=indexing
                      tunnel: [w247] -> w235 mode=indexing
                      n63 = call-poly <vilib>:"Append Digital Samples.vi"("digital waveform B"=w248, "digital waveform A"=w249) -> ("digital waveform out"=w247:digitalwaveform)  [unwired: 8 in, 1 out]
                    }
                    n64 = for {
                      tunnel: w238 -> [w251] mode=indexing
                      tunnel: w239 -> [w252] mode=indexing
                      tunnel: [w250] -> w237 mode=indexing
                      n65 = call-poly <vilib>:"Append Waveforms.vi"("waveform B"=w251, "waveform A"=w252) -> ("waveform out"=w250:waveform(dbl))  [unwired: 8 in, 1 out]
                    }
                  }
                  n66 = Bundle(w222, w226) -> (w223:cluster{waveform(dbl)[], digitalwaveform[]})  [unwired: 1 in]
                }
                frame "XYZT" {
                }
                frame "XYZC" {
                }
              }
              n67 = call "Graph.vi"("Cluster"=w194) -> ()
            }
            frame "runWaves" {
              n68 = Unbundle By Name(w289) -> ("Samples per millisecond"=w261:dbl)
              n69 = Index Array(array=w288, index=0) -> (element=w286:waveform(dbl))
              n70 = Multiply(x=w261, y=1000.0) -> (x*y=w281:dbl)
              n71 = local read "Scan Continuously"() -> (w282:bool)
              n72 = call-poly <vilib>:"Number of Waveform Samples.vi"("waveform in"=w286) -> ("number of samples"=w262:i32)  [unwired: 8 in, 2 out]
              n73 = call-poly <vilib>:"DAQmx Timing.vi"("task/channels in"=w291, "samples per channel"=w262, "rate"=w281, "error in"=w264) -> ("task out"=w294:refnum<k21>, "error out"=w285:errorcluster)  [unwired: 10 in]
              n74 = call-poly <vilib>:"DAQmx Timing.vi"("task/channels in"=w279, "samples per channel"=w262, "rate"=w281, "error in"=w264) -> ("task out"=w280:refnum<k21>, "error out"=w277:errorcluster)  [unwired: 10 in]
              n75 = case shown="True" w282 {
                tunnel: w290 -> [w296 w304]
                tunnel: [w297 w303] -> _
                tunnel: w289 -> [w298 w302]
                frame False {
                  n76 = Bundle("Mode"=ModeEnum."Idle", "Microscope Settings"=w298) -> (w299:cluster{"Mode":T7, "Microscope Settings":T1})  [unwired: 1 in]
                  n77 = Enqueue Element(queue=w296, element=w299) -> (queue out=w297:refnum<queue>)  [unwired: 2 in, 2 out]
                }
                frame True {
                  n78 = Bundle("Mode"=ModeEnum."runWaves", "Microscope Settings"=w302) -> (w301:cluster{"Mode":T7, "Microscope Settings":T1})  [unwired: 1 in]
                  n79 = Enqueue Element(queue=w304, element=w301) -> (queue out=w303:refnum<queue>)  [unwired: 2 in, 2 out]
                }
              }
              n80 = call-poly <vilib>:"DAQmx Write.vi"("task/channels in"=w294, "data"=w288, "error in"=w285) -> ("task out"=w272:refnum<k21>, "error out"=w275:errorcluster)  [unwired: 10 in, 1 out]
              n81 = call-poly <vilib>:"DAQmx Write.vi"("task/channels in"=w280, "data"=w270, "error in"=w277) -> ("task out"=w271:refnum<k21>, "error out"=w274:errorcluster)  [unwired: 10 in, 1 out]
              n82 = Merge Errors(w275, w274) -> (w273:errorcluster)
              n83 = call <vilib>:"DAQmx Start Task.vi"("task/channels in"=w272, "error in"=w273) -> ("task out"=w293:refnum<k21>, "error out"=w292:errorcluster)  [unwired: 12 in]
              n84 = call <vilib>:"DAQmx Start Task.vi"("task/channels in"=w271, "error in"=w273) -> ("task out"=w278:refnum<k21>, "error out"=w276:errorcluster)  [unwired: 12 in]
              n85 = call <vilib>:"DAQmx Wait Until Done.vi"("task/channels in"=w293, "error in"=w292) -> ("task out"=w284:refnum<k21>, "error out"=w267:errorcluster)  [unwired: 12 in]
              n86 = call <vilib>:"DAQmx Wait Until Done.vi"("task/channels in"=w278, "error in"=w276) -> ("task out"=w269:refnum<k21>, "error out"=w266:errorcluster)  [unwired: 12 in]
              n87 = call <vilib>:"DAQmx Stop Task.vi"("task/channels in"=w284) -> ("task out"=w283:refnum<k21>)  [unwired: 13 in, 1 out]
              n88 = Merge Errors(w267, w266) -> (w265:errorcluster)
              n89 = call <vilib>:"DAQmx Stop Task.vi"("task/channels in"=w269) -> ("task out"=w268:refnum<k21>)  [unwired: 13 in, 1 out]
            }
            frame "stop" {
            }
          }
          n90 = local read "stop"() -> (w170:bool)
          n91 = Or(x=w171, y=w170) -> (x .or. y?=w169:bool)
        }
        n92 = while {
          tunnel: w153 -> [w530]
          shift-right: [w529] -> _
          shift-left: _ -> [w528]
          tunnel: w145 -> [w526]
          shift-right: [w525] -> _
          shift-left: w142 -> [w524]
          stop <- w531 stop-if-true
          n93 = event shown="[5] \"Microscope Settings.Piezo Position /um\": Value Change" {
            selector: _ -> [_ _ _ _ _ _ _ _ _ _ _]
            dyn-events: _ -> [_ _ _ _ _ _ _ _ _ _ _]
            timeout: 1 -> [_ _ _ _ _ _ _ _ _ _ _]
            tunnel: [w540 _ _ _ _ _ _ _ _ _ _] -> w531
            tunnel: w530 -> [w535 _ w554 w559 w566 _ _ w581 _ _ _]
            tunnel: [w533 _ w548 w557 _ _ _ _ _ _ w608] -> w529
            tunnel: w528 -> [w533 w546 w548 w557 w562 w569 w576 w582 _ w596 _]
            tunnel: [_ _ _ w558 _ _ _ _ _ w595 _] -> _
            tunnel: w526 -> [w534 _ w553 w558 w563 w570 w575 w580 _ w594 _]
            tunnel: [w532 w541 w547 w555 w565 w573 w574 w579 w588 w592 w607] -> w525
            tunnel: w524 -> [w532 w543 w547 w555 w565 w573 w574 w579 w588 w592 w607]
            event "stop": Value Change {
              w538 = ModeEnum."stop"  # Mode
              n94 = event-data() -> ()  [unwired: 1 in, 6 out]
              n95 = Bundle("Enum"=CameraControlTypeDef."Idle", "Value"=w533) -> (w536:cluster{"Enum":T8, "Value":T1})  [unwired: 1 in]
              n96 = Bundle("Mode"=w538, "Value"=w533) -> (w537:cluster{"Mode":T7, "Value":T1})  [unwired: 1 in]
              n97 = Enqueue Element(queue=w535, element=w536) -> ()  [unwired: 2 in, 3 out]
              n98 = Enqueue Element(queue=w534, element=w537) -> ()  [unwired: 2 in, 3 out]
              n99 = local read "stop"() -> (w540:bool)
            }
            event Value Change {
              n100 = event-data() -> ()  [unwired: 1 in, 6 out]
              n101 = Flatten To XML(anything=w546) -> (xml string=w545:string)
              n102 = Build Array("Experiment 1" ("element"), w545) -> (w542:string[])
              n103 = Build Array (concatenate)(w543, w542) -> (w541:string[][])
              n104 = property on="Multicolumn Listbox" class="MCListbox (strict)"("ItemNames"=w541) -> ()  [unwired: 2 in, 2 out]
            }
            event Value Change {
              w551 = ModeEnum."generateWaves"  # Mode
              # "Live video for Calibration and 2D\nScan Modes.\n\nIdle Video for MultiD Scan modes\nUNTIL Begin Scan Button pressed?\n\nMultiD is waiting for trigger"
              n105 = event-data() -> ()  [unwired: 1 in, 6 out]
              n106 = Bundle("Enum"=CameraControlTypeDef."Trigger Source", "Value"=w548) -> (w549:cluster{"Enum":T8, "Value":T1})  [unwired: 1 in]
              n107 = Bundle("Mode"=w551, "Value"=w548) -> (w550:cluster{"Mode":T7, "Value":T1})  [unwired: 1 in]
              n108 = Enqueue Element(queue=w554, element=w549) -> ()  [unwired: 2 in, 3 out]
              n109 = Enqueue Element(queue=w553, element=w550) -> ()  [unwired: 2 in, 3 out]
            }
            event Value Change {
              n110 = event-data() -> ()  [unwired: 1 in, 6 out]
              n111 = Bundle("Enum"=CameraControlTypeDef."Readout Mode", "Value"=w557) -> (w556:cluster{"Enum":T8, "Value":T1})  [unwired: 1 in]
              n112 = Enqueue Element(queue=w559, element=w556) -> ()  [unwired: 2 in, 3 out]
            }
            event Value Change {
              w561 = ModeEnum."generateWaves"  # Mode
              n113 = event-data() -> ()  [unwired: 1 in, 6 out]
              n114 = Bundle("Enum"=CameraControlTypeDef."ROI", "Value"=w562) -> (w567:cluster{"Enum":T8, "Value":T1})  [unwired: 1 in]
              n115 = Bundle("Mode"=w561, "Value"=w562) -> (w564:cluster{"Mode":T7, "Value":T1})  [unwired: 1 in]
              n116 = Enqueue Element(queue=w566, element=w567) -> ()  [unwired: 2 in, 3 out]
              n117 = Enqueue Element(queue=w563, element=w564) -> ()  [unwired: 2 in, 3 out]
            }
            event Value Change {
              w571 = ModeEnum."generateWaves"  # Mode
              n118 = event-data() -> ()  [unwired: 1 in, 6 out]
              n119 = Bundle("Mode"=w571, "Value"=w569) -> (w572:cluster{"Mode":T7, "Value":T1})  [unwired: 1 in]
              n120 = Enqueue Element(queue=w570, element=w572) -> ()  [unwired: 2 in, 3 out]
            }
            event Value Change {
              w578 = ModeEnum."generateWaves"  # Mode
              n121 = event-data() -> ()  [unwired: 1 in, 6 out]
              n122 = Bundle("Mode"=w578, "Value"=w576) -> (w577:cluster{"Mode":T7, "Value":T1})  [unwired: 1 in]
              n123 = Enqueue Element(queue=w575, element=w577) -> ()  [unwired: 2 in, 3 out]
            }
            event Value Change {
              w585 = ModeEnum."generateWaves"  # Mode
              n124 = event-data() -> ()  [unwired: 1 in, 6 out]
              n125 = Bundle("Enum"=CameraControlTypeDef."Update", "Value"=w582) -> (w583:cluster{"Enum":T8, "Value":T1})  [unwired: 1 in]
              n126 = Bundle("Mode"=w585, "Value"=w582) -> (w584:cluster{"Mode":T7, "Value":T1})  [unwired: 1 in]
              n127 = Enqueue Element(queue=w581, element=w583) -> ()  [unwired: 2 in, 3 out]
              n128 = Enqueue Element(queue=w580, element=w584) -> ()  [unwired: 2 in, 3 out]
            }
            event "Signals Debugger": Value Change {
              n129 = event-data() -> ()  [unwired: 1 in, 6 out]
              n130 = case shown="True" "Signals Debugger" {
                frame False {
                }
                frame True {
                  n131 = vi-ref "Graph.vi"() -> (w589:refnum<vi>)
                  n132 = invoke class="VI" method="FP.Open"(reference=w589, "Activate"=TRUE ("Front Panel Window:Open"), "State"=T12."Standard") -> ()  [unwired: 2 in, 5 out]
                }
              }
            }
            event "Scan": Value Change {
              n133 = event-data() -> ("NewVal"=w593:bool)  [unwired: 1 in, 5 out]
              n134 = case shown="True" w593 {
                tunnel: w596 -> [_ w601]
                tunnel: [w597 w600] -> w595
                tunnel: w594 -> [w597 w599]
                frame False {
                }
                frame True {
                  n135 = for {
                    N: "Scans" -> [_]
                    tunnel: w601 -> [w603]
                    tunnel: [w602] -> w600
                    tunnel: w599 -> [w606]
                    w605 = ModeEnum."runWaves"  # Mode
                    n136 = Bundle("Mode"=w605, "Value"=w603) -> (w604:cluster{"Mode":T7, "Value":T1})  [unwired: 1 in]
                    n137 = Enqueue Element(queue=w606, element=w604) -> (queue out=w602:refnum<queue>)  [unwired: 2 in, 2 out]
                  }
                }
              }
            }
            event Timeout {
              n138 = event-data() -> ()  [unwired: 1 in, 3 out]
              n139 = property on="Microscope Settings" class="Clust (strict)"() -> ("Value"=w608:T1)  [unwired: 2 in, 2 out]
            }
          }
        }
        n140 = while "Camera Consumer" {
          tunnel: w160 -> [w352]
          tunnel: [w337] -> w164
          tunnel: w153 -> [w345]
          tunnel: [w353] -> w163
          shift-right: [w351] -> _
          shift-left: CameraControlTypeDef."Preview" ("Enum") -> [w341]
          tunnel: [w348] -> w158
          tunnel: w157 -> [w347]
          tunnel: w155 -> [w340]
          shift-right: [w349] -> w167
          shift-left: w168 -> [w350]
          stop <- w336 stop-if-true
          n141 = Dequeue Element(queue=w345, timeout in ms (-1)=1) -> (queue out=w344:refnum<queue>, element=w339:cluster{"Enum":T8, "Microscope Settings":T1}, timed out?=w343:bool)  [unwired: 1 in, 1 out]
          n142 = case shown="True" w343 {
            tunnel: [w355 CameraControlTypeDef."Preview" ("Enum")] -> w342
            tunnel: w341 -> [_ _]
            tunnel: w339 -> [w356 _]
            tunnel: [w354 _] -> w338
            frame False {
              n143 = Unbundle(w356) -> ("Enum"=w355:T8, "Microscope Settings"=w354:T1)
            }
            frame True {
            }
          }
          n144 = case shown="\"Readout Mode\"" w342 {
            selector: w342 -> [w361 w366 w371 w376 w381 w392 w397 w402 w407 w412 w445 w463 _ w492 _]
            tunnel: w344 -> [w360 w367 w372 w377 w382 w393 w398 w403 w408 w413 _ w459 w474 w494 w513]
            tunnel: [w360 w367 w372 w377 w382 w393 w398 w403 w408 w413 _ w459 w474 w494 w513] -> w353
            tunnel: w352 -> [w362 w365 w370 w375 w380 w391 w396 w401 w406 w411 w440 w462 w466 w491 w504]
            tunnel: [w362 w365 w370 w375 w380 w391 w396 w401 w406 w411 w414 w462 w465 w491 w505] -> w337
            tunnel: [w361 w366 w371 w376 w381 w392 w397 w402 w407 w412 w445 w463 CameraControlTypeDef."Preview" ("Enum") w492 w495] -> w351
            tunnel: w350 -> [w359 w364 w369 w374 w378 w389 w395 w400 w405 w410 w442 w461 w472 w493 w507]
            tunnel: [w359 w364 w369 w374 w378 w388 w395 w400 w405 w410 w416 w461 w470 w493 w506] -> w349
            tunnel: [w358 w363 w368 w373 w379 w390 w394 w399 w404 w409 w444 w460 w468 w490 w508] -> w348
            tunnel: w347 -> [w358 w363 w368 w373 w379 w390 w394 w399 w404 w409 w444 w460 w468 w490 _]
            tunnel: w340 -> [_ _ _ _ _ _ _ _ _ _ _ _ w467 _ _]
            tunnel: w338 -> [_ _ _ _ _ w387 _ _ _ _ w439 _ _ _ w497]
            frame "Idle" {
            }
            frame "IntervalLineInt" {
            }
            frame "Ram Record" {
            }
            frame "HardDisk Record" {
            }
            frame "Disengage Update" {
            }
            frame "Update", Default {
              w384 = u32 2049184 items=["SENSOR MODE"=4212128, "CCD MODE"=4212384, "READOUT MODE"=4211872, "ACTIVE VIEW INDEX"=4343136, "BITS PER CHANNEL"=4342976, "IMAGE PIXEL TYPE"=4343296, "BINNING"=4215968, "EXPOSURE TIME"=2049184, "CONTRAST GAIN"=3163312, "CONTRAST OFFSET"=3163328, "LIGHT MODE"=2114720, "SENSITIVITY"=2114992, "PHOTON IMAGING MODE"=2115200, "HIGH DYNAMIC RANGE MODE"=3163360, "WHITE BALANCE"=3163568, "TEMPERATURE"=2115232, "TEMPERATURE TARGET"=2115264, "SENSOR COOLER FAN"=2115296, "LINEBUNDLE HEIGHT"=4212192, "MECHANICAL SHUTTER"=2115488, "BACK FOCUS POSITION"=8422304, "TRIGGER CONNECTOR"=1066432, "TRIGGER SOURCE"=1066144, "OUTPUT TRIGGER SOURCE"=1852576, "TRIGGER GLOBAL EXPOSURE"=2049680, "FIRST TRIGGER BEHAVIOR"=2049696, "CHANNEL SYNC"=1852352, "READOUT DIRECTION"=4211904, "PRE HSYNC COUNT"=1852704, "INTERNAL LINE SPEED"=4226000, "INTERNAL LINE INTERVAL"=4226016] ("Parameter")
              n145 = Unbundle By Name(w387) -> ("Exposure/ms"=w386:dbl)  [unwired: 1 out]
              n146 = Divide(x=w386, y=1000.0) -> (x/y=w383:dbl)
              n147 = call "tm_setparameter_a.vi"("Value in"=w383, "Parameter"=w384, "Handle in"=w389) -> ("Handle out"=w388:u32)  [unwired: 7 in, 1 out]
            }
            frame "ROI" {
            }
            frame "Binning" {
            }
            frame "Scan Mode" {
            }
            frame "Trigger Mode" {
            }
            frame "Readout Mode" {
              w420 = 1 items=["Snap", "Sequence"] ("Capture mode")
              w426 = u32 4194832  # Sensor Mode
              w429 = u32 2031888  # Exposure time
              n148 = Unbundle By Name(w439) -> ("Exposure/ms"=w438:dbl, "Slit.Slit Width /%"=w434:dbl, "Slit.Scanning Mode"=w424:dbl)
              n149 = call "tm_stopcapture.vi"("error in (no error)"=w440, "Handle in"=w442) -> ("error out"=w443:errorcluster, "Handle out"=w441:u32)  [unwired: 8 in]
              n150 = Divide(x=w438, y=1000.0) -> (x/y=w436:dbl)
              n151 = Multiply(x=w434, y=2048 ("input variable")) -> (x*y=w433:dbl)
              n152 = call "tm_unpreparecapture.vi"("error in (no error)"=w443, "Handle in"=w441) -> ("error out"=w421:errorcluster, "Handle out"=w425:u32)  [unwired: 8 in]
              n153 = call "tm_setpropertyvalue.vi"("error in (no error)"=w421, "Value in"=w424, "Property ID"=w426, "Handle in"=w425) -> ("error out"=w422:errorcluster, "Handle out"=w423:u32)  [unwired: 6 in]
              n154 = Divide(x=w433, y=100.0) -> (x/y=w431:dbl)
              n155 = case shown="1, Default" w424 {
                tunnel: [w448 w449] -> w430
                tunnel: w436 -> [w448 w457]
                tunnel: w431 -> [_ w456]
                tunnel: w423 -> [w447 w451]
                tunnel: [w447 w453] -> w428
                tunnel: [w446 w452] -> w427
                tunnel: w422 -> [w446 w450]
                frame 1, Default {
                }
                frame 12 {
                  w455 = u32 4208720  # Line Interval
                  n156 = formula code="slitExpos=frameInter*LW/(LinesToReadout\n+10+LW);\nlineInter = slitExpos / LW;"("frameInter"=w457, "LW"=w456, "LinesToReadout"=2048 ("input variable")) -> ("slitExpos"=w449:dbl, "lineInter"=w454:dbl)
                  n157 = call "tm_setpropertyvalue.vi"("error in (no error)"=w450, "Value in"=w454, "Property ID"=w455, "Handle in"=w451) -> ("error out"=w452:errorcluster, "Handle out"=w453:u32)  [unwired: 6 in]
                }
              }
              n158 = call "tm_setpropertyvalue.vi"("error in (no error)"=w427, "Value in"=w430, "Property ID"=w429, "Handle in"=w428) -> ("error out"=w415:errorcluster, "Handle out"=w417:u32)  [unwired: 6 in]
              n159 = call "tm_preparecapture.vi"("error in (no error)"=w415, "Capture mode"=w420, "Handle in"=w417) -> ("error out"=w419:errorcluster, "Handle out"=w418:u32)  [unwired: 5 in, 2 out]
              n160 = call "tm_startcapture_b.vi"("error in (no error)"=w419, "Handle in"=w418) -> ("error out"=w414:errorcluster, "Handle out"=w416:u32)  [unwired: 8 in]
            }
            frame "Readout Direction" {
            }
            frame "Preview" {
              n161 = call "tm_waitnextframe.vi"("error in (no error)"=w466, "Timeout"=500, "Handle in"=w472) -> ("error out"=w464:errorcluster, "Handle out"=w471:u32)  [unwired: 5 in, 2 out]
              n162 = case shown="No Error" w464 {
                selector: w464 -> [w475 w489]
                tunnel: w471 -> [w487 w488]
                tunnel: [w486 w488] -> w470
                tunnel: w468 -> [w485 _]
                tunnel: w467 -> [w484 _]
                tunnel: w466 -> [w479 _]
                tunnel: [w476 w489] -> w465
                frame No Error {
                  w481 = 0 ("Timeout")
                  n163 = call "tm_getframe_a.vi"("error in (no error)"=w475, "Buffer Info"=w485, "Handle in"=w487) -> ("error out"=w477:errorcluster, "Data 16"=w482:u16[][], "Handle out"=w486:u32)  [unwired: 4 in, 2 out]
                  n164 = Bundle("State"=Stack_Track."Display", "Timeout"=w481, "Data 16"=w482, "Timeout"=w481) -> (w480:T15)  [unwired: 1 in]
                  n165 = Enqueue Element(queue=w484, element=w480, error in (no error)=w479) -> (error out=w478:errorcluster)  [unwired: 1 in, 2 out]
                  n166 = Merge Errors(w477, w478) -> (w476:errorcluster)
                }
                frame Error {
                }
              }
            }
            frame "ROIWindow" {
            }
            frame "Trigger Source" {
              (unwired) u32 1066144 items=["SENSOR MODE"=4212128, "CCD MODE"=4212384, "READOUT MODE"=4211872, "ACTIVE VIEW INDEX"=4343136, "BITS PER CHANNEL"=4342976, "IMAGE PIXEL TYPE"=4343296, "BINNING"=4215968, "EXPOSURE TIME"=2049184, "CONTRAST GAIN"=3163312, "CONTRAST OFFSET"=3163328, "LIGHT MODE"=2114720, "SENSITIVITY"=2114992, "PHOTON IMAGING MODE"=2115200, "HIGH DYNAMIC RANGE MODE"=3163360, "WHITE BALANCE"=3163568, "TEMPERATURE"=2115232, "TEMPERATURE TARGET"=2115264, "SENSOR COOLER FAN"=2115296, "LINEBUNDLE HEIGHT"=4212192, "MECHANICAL SHUTTER"=2115488, "BACK FOCUS POSITION"=8422304, "TRIGGER CONNECTOR"=1066432, "TRIGGER SOURCE"=1066144, "OUTPUT TRIGGER SOURCE"=1852576, "TRIGGER GLOBAL EXPOSURE"=2049680, "FIRST TRIGGER BEHAVIOR"=2049696, "CHANNEL SYNC"=1852352, "READOUT DIRECTION"=4211904, "PRE HSYNC COUNT"=1852704, "INTERNAL LINE SPEED"=4226000, "INTERNAL LINE INTERVAL"=4226016] ("Parameter")
              w503 = 1 items=["Snap", "Sequence"] ("Capture mode")
              n167 = Unbundle By Name(w497) -> ("Mode"=w496:enum16{"X", "XY", "XYZ", "XYZT", "XYZC"})
              n168 = call "tm_stopcapture.vi"("error in (no error)"=w504, "Handle in"=w507) -> ("error out"=w511:errorcluster, "Handle out"=w512:u32)  [unwired: 8 in]
              n169 = call "tm_unpreparecapture.vi"("error in (no error)"=w511, "Handle in"=w512) -> ("error out"=w499:errorcluster, "Handle out"=w502:u32)  [unwired: 8 in]
              n170 = case shown="\"XYZT\"" w496 {
                tunnel: [T9 {"Mode"=2, "Polarity"=2, "Times"=2, "Delay"=0.0} ("Parameters") T9 {"Mode"=2, "Polarity"=2, "Times"=2, "Delay"=0.0} ("Parameters") T9 {"Mode"=2, "Polarity"=2, "Times"=2, "Delay"=0.0} ("Parameters") T9 {"Mode"=1, "Polarity"=2, "Times"=2, "Delay"=0.0} ("Parameters") T9 {"Mode"=1, "Polarity"=2, "Times"=2, "Delay"=0.0} ("Parameters")] -> w500
                tunnel: [CameraControlTypeDef."Preview" ("Enum") CameraControlTypeDef."Idle" ("Enum") CameraControlTypeDef."Idle" ("Enum") CameraControlTypeDef."Idle" ("Enum") CameraControlTypeDef."Preview" ("Enum")] -> w495
                frame "XY", Default {
                }
                frame "XYZT" {
                }
                frame "XYZ" {
                }
                frame "XYZC" {
                }
                frame "X" {
                }
              }
              n171 = call <userlib>:"tm_setinputtrigger.vi"("error in (no error)"=w499, "Parameters"=w500, "Handle in"=w502) -> ("error out"=w498:errorcluster, "Handle out"=w501:u32)  [unwired: 7 in]
              n172 = call "tm_preparecapture.vi"("error in (no error)"=w498, "Capture mode"=w503, "Handle in"=w501) -> ("error out"=w510:errorcluster, "Buffer Info"=w508:T5, "Handle out"=w509:u32)  [unwired: 5 in, 1 out]
              n173 = call "tm_startcapture_b.vi"("error in (no error)"=w510, "Handle in"=w509) -> ("error out"=w505:errorcluster, "Handle out"=w506:u32)  [unwired: 8 in]
            }
          }
          n174 = local read "stop"() -> (w336:bool)
        }
        n175 = while "Tiff Consumer" {
          tunnel: [w314] -> w165
          tunnel: [w317] -> w162
          tunnel: w155 -> [w319]
          tunnel: w154 -> [w311]
          stop <- w321 stop-if-true
          # "Delay, maybe?\nCheck"
          n176 = Dequeue Element(queue=w319, timeout in ms (-1)=1) -> (queue out=w316:refnum<queue>, element=w318:T10, error out=w315:errorcluster)  [unwired: 1 in, 1 out]
          n177 = Unbundle By Name(w318) -> ("State"=w312:T11, "Image"=w313:u16[][])  [unwired: 1 out]
          n178 = case shown="\"Idle\", Default" w312 {
            selector: w312 -> [_ w332 w333]
            tunnel: [w329 w331 w334] -> w317
            tunnel: w316 -> [w329 w331 w334]
            tunnel: [Stack_Track."Idle" ("State") w332 w333] -> _
            tunnel: w313 -> [w324 _ _]
            tunnel: w311 -> [w328 _ _]
            tunnel: w315 -> [w327 w330 w335]
            tunnel: [w326 w330 w335] -> w314
            frame "Display" {
              n179 = call "IMAQ ArrayToImage"("Image Pixels (U16)"=w324, "error in (no error)"=w327, "Image"=w328) -> ("error out"=w326:errorcluster, "Image Out"=w323:T3)  [unwired: 7 in]
              "Image" <- w323
              n180 = call "IMAQ Histograph"("Image"=w323) -> ("Histogram Graph"=→"Histogram":T4)  [unwired: 7 in, 3 out]
            }
            frame "Idle", Default {
            }
            frame "Start Sequence" {
            }
          }
          n181 = local read "stop"() -> (w321:bool)
        }
        n182 = Merge Errors(w164, w165, w143) -> (w166:errorcluster)
      }
      frame "deinit" {
        n183 = call <vilib>:"DAQmx Stop Task.vi"("task/channels in"=w619) -> ("task out"=w620:refnum<k21>)  [unwired: 13 in, 1 out]
        n184 = call <vilib>:"DAQmx Stop Task.vi"("task/channels in"=w621) -> ("task out"=w622:refnum<k21>)  [unwired: 13 in, 1 out]
        n185 = call <vilib>:"DAQmx Clear Task.vi"("task in"=w620) -> ("error out"=w616:errorcluster)  [unwired: 14 in]
        n186 = call "tm_stopcapture.vi"("error in (no error)"=w631, "Handle in"=w627) -> ("error out"=w634:errorcluster, "Handle out"=w633:u32)  [unwired: 8 in]
        n187 = call <vilib>:"DAQmx Clear Task.vi"("task in"=w622) -> ("error out"=w617:errorcluster)  [unwired: 14 in]
        n188 = call "tm_unpreparecapture.vi"("error in (no error)"=w634, "Handle in"=w633) -> ("error out"=w635:errorcluster, "Handle out"=w632:u32)  [unwired: 8 in]
        n189 = call "tm_closecamera.vi"("error in (no error)"=w635, "Handle in"=w632) -> ("error out"=w636:errorcluster)  [unwired: 9 in]
        n190 = Flush Queue(queue=w609) -> (queue out=w615:refnum<queue>)  [unwired: 1 in, 2 out]
        n191 = call "tm_deinitialize.vi"("error in (no error)"=w636) -> ("error out"=w612:errorcluster)  [unwired: 10 in]
        n192 = Release Queue(queue=w610, error in (no error)=w612) -> (error out=w629:errorcluster)  [unwired: 1 in, 2 out]
        n193 = Release Queue(queue=w615) -> (error out=w618:errorcluster)  [unwired: 2 in, 2 out]
        n194 = Flush Queue(queue=w614, error in (no error)=w612) -> (queue out=w613:refnum<queue>, error out=w611:errorcluster)  [unwired: 1 out]
        n195 = Release Queue(queue=w613, error in (no error)=w611) -> (error out=w628:errorcluster)  [unwired: 1 in, 2 out]
        n196 = Merge Errors(w629, w628, w618, w617, w616) -> (w630:errorcluster)
      }
    }
    n197 = Or(x="stop", y=w17) -> (x .or. y?=w18:bool)
  }
  "error IO" <- w5
  n198 = disable-structure shown="Enabled" {
    frame Disabled {
      # "Parallise decode buffer"
      n199 = call "tm_startcapture_b.vi"() -> ()  [unwired: 10 in, 2 out]
      n200 = call "tm_waitnextframe.vi"() -> ()  [unwired: 8 in, 4 out]
      n201 = call "tm_getframe_a.vi"() -> ()  [unwired: 7 in, 5 out]
    }
    frame Enabled {
    }
  }
